vi "SP1461.vi"(1 "Port":refnum<visa-resource-name>, 2 "In":variant, 3 "Mode":u32(ring) items=["Open", "Close", "Begin", "End", "Get", "Set"]) -> (0 "Out":variant)   [LabVIEW 2014]
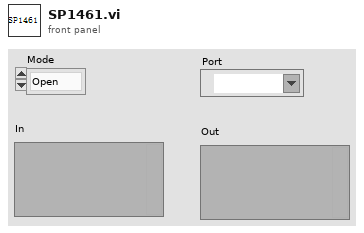
[diagram p1: front panel]
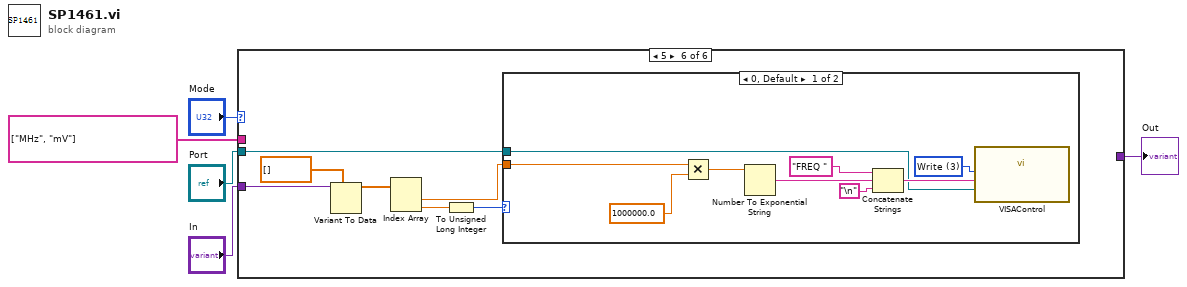
[diagram p0: block diagram]
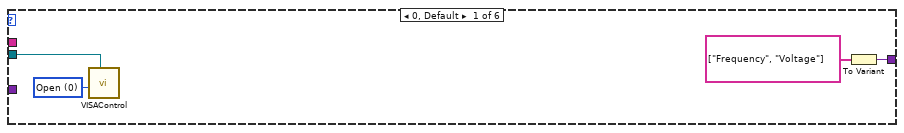
[diagram p2: hidden frame]
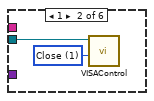
[diagram p3: hidden frame]
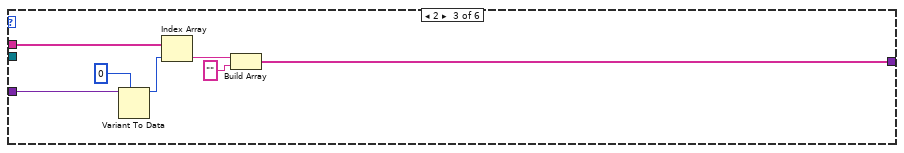
[diagram p4: hidden frame]
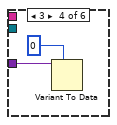
[diagram p5: hidden frame]
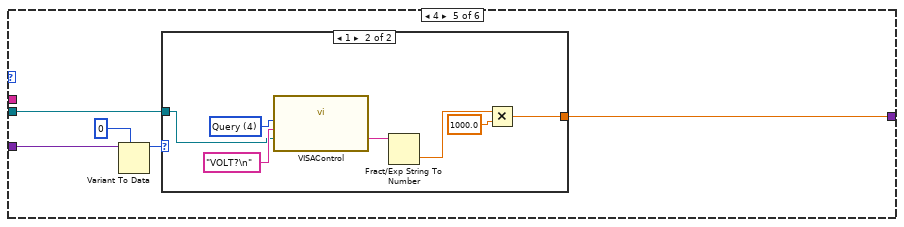
[diagram p6: hidden frame]
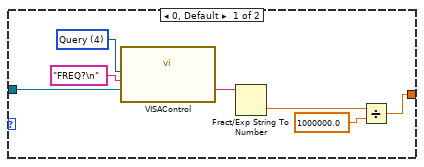
[diagram p7: hidden frame]
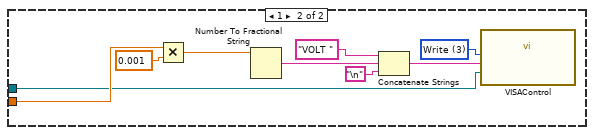
[diagram p8: hidden frame]
diagram:
  n1 = case shown="5" "Mode" {
    tunnel: "In" -> [_ _ w18 w19 w24 w45]
    tunnel: [w8 _ w12 _ w21 _] -> w3
    tunnel: "Port" -> [w6 w10 _ _ w22 w40]
    tunnel: string[] ["MHz", "mV"] ("Strings []") -> [_ _ w15 _ _ _]
    frame 0, Default {
      w7 = u32 0 items=["Open", "Close", "Read", "Write", "Query"] ("Mode")
      n2 = call "VISAControl.vi"("Mode"=w7, "Name"=w6) -> ()  [unwired: 3 in, 2 out]
      n3 = To Variant(anything=string[] ["Frequency", "Voltage"] ("Strings []")) -> (Variant=w8:variant)
    }
    frame 1 {
      w11 = u32 1 items=["Open", "Close", "Read", "Write", "Query"] ("Mode")
      n4 = call "VISAControl.vi"("VISA in"=w10, "Mode"=w11) -> ()  [unwired: 3 in, 2 out]
    }
    frame 2 {
      n5 = Variant To Data(type=0, Variant=w18) -> (data=w14:i32)  [unwired: 1 in, 1 out]
      n6 = Index Array(array=w15, index=w14) -> (element=w13:string)
      n7 = Build Array(w13, "") -> (w12:string[])
    }
    frame 3 {
      n8 = Variant To Data(type=0, Variant=w19) -> ()  [unwired: 1 in, 2 out]
    }
    frame 4 {
      n9 = Variant To Data(type=u32 0, Variant=w24) -> (data=w23:u32)  [unwired: 1 in, 1 out]
      n10 = case shown="1" w23 {
        tunnel: w22 -> [w26 w33]
        tunnel: [w27 w34] -> w21
        frame 0, Default {
          w31 = u32 4 items=["Open", "Close", "Read", "Write", "Query"] ("Mode")
          n11 = call "VISAControl.vi"("Mode"=w31, "Write Buffer"="FREQ?\n", "Name"=w26) -> ("Read Buffer"=w29:string)  [unwired: 2 in, 1 out]
          n12 = Fract/Exp String To Number(string=w29) -> (number=w28:dbl)  [unwired: 3 in, 1 out]
          n13 = Divide(x=w28, y=1000000.0) -> (x/y=w27:dbl)
        }
        frame 1 {
          w39 = u32 4 items=["Open", "Close", "Read", "Write", "Query"] ("Mode")
          n14 = call "VISAControl.vi"("Mode"=w39, "Write Buffer"="VOLT?\n", "Name"=w33) -> ("Read Buffer"=w38:string)  [unwired: 2 in, 1 out]
          n15 = Fract/Exp String To Number(string=w38) -> (number=w35:dbl)  [unwired: 3 in, 1 out]
          n16 = Multiply(x=w35, y=1000.0) -> (x*y=w34:dbl)
        }
      }
    }
    frame 5 {
      n17 = Variant To Data(type=dbl[] [] ("appended array"), Variant=w45) -> (data=w44:dbl[])  [unwired: 1 in, 1 out]
      n18 = Index Array(array=w44) -> (element #1=w41:dbl, element #2=w43:dbl)  [unwired: 2 in]
      n19 = To Unsigned Long Integer(number=w43) -> (unsigned 32bit integer=w42:u32)
      n20 = case shown="0, Default" w42 {
        tunnel: w41 -> [w48 w57]
        tunnel: w40 -> [w47 w56]
        frame 0, Default {
          w54 = u32 3 items=["Open", "Close", "Read", "Write", "Query"] ("Mode")
          n21 = Multiply(x=w48, y=1000000.0) -> (x*y=w50:dbl)
          n22 = Number To Exponential String(number=w50) -> (E-format string=w49:string)  [unwired: 3 in]
          n23 = Concatenate Strings("FREQ " ("Write Buffer"), w49, "\n") -> (w52:string)
          n24 = call "VISAControl.vi"("Mode"=w54, "Write Buffer"=w52, "Name"=w47) -> ()  [unwired: 2 in, 2 out]
        }
        frame 1 {
          w64 = u32 3 items=["Open", "Close", "Read", "Write", "Query"] ("Mode")
          n25 = Multiply(x=w57, y=0.001) -> (x*y=w58:dbl)
          n26 = Number To Fractional String(number=w58) -> (F-format string=w61:string)  [unwired: 3 in]
          n27 = Concatenate Strings("VOLT " ("Write Buffer"), w61, "\n") -> (w62:string)
          n28 = call "VISAControl.vi"("Mode"=w64, "Write Buffer"=w62, "Name"=w56) -> ()  [unwired: 2 in, 2 out]
        }
      }
    }
  }
  "Out" <- w3
